vi "Hertz Timer.vi"(11 "How many times per second do we want the loop to run?":i32=100) -> ()   [LabVIEW 2012]
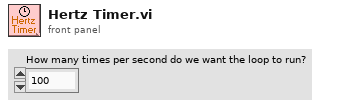
[diagram p1: front panel]
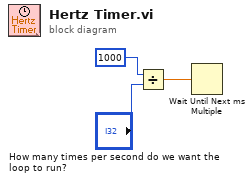
[diagram p0: block diagram]
diagram:
  n1 = Divide(x=1000, y="How many times per second do we want the loop to run?") -> (x/y=w3:dbl)
  n2 = Wait Until Next ms Multiple(millisecond multiple=w3) -> ()  [unwired: 1 out]
